vi "SPD.Get Meas pass and report.vi"(8 "error in (no error)":errorcluster, 11 "error or stoped":bool) -> (0 "error out":errorcluster, 2 "pass":bool, 3 "report":string)   [LabVIEW 2018]
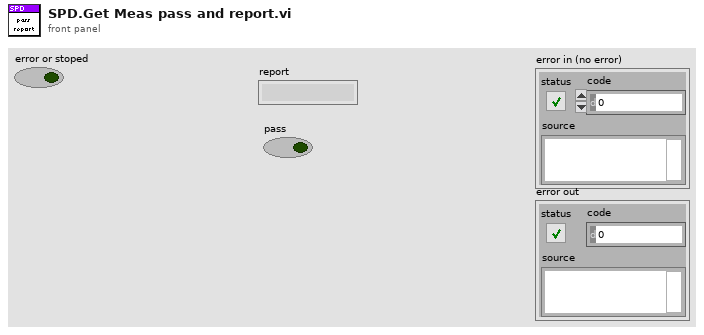
[diagram p1: front panel]
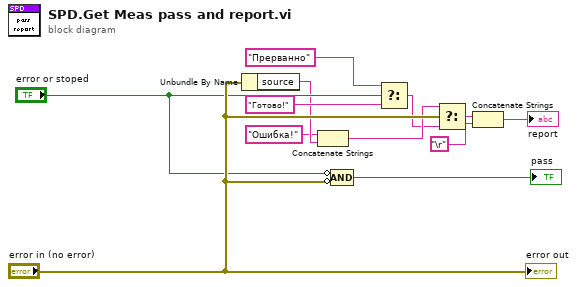
[diagram p0: block diagram]
diagram:
  n1 = Unbundle By Name("error in (no error)") -> ("source"=w5:string)
  n2 = Concatenate Strings("Ошибка!" ("t"), w5) -> (w4:string)
  n3 = Compound Arithmetic op=AND(invert "error or stoped", invert "error in (no error)") -> (→"pass":bool)
  n4 = Select(t="Прерванно" ("Report"), s="error or stoped", f="Готово!") -> (s? t:f=w2:string)
  n5 = Select(t=w4, s="error in (no error)", f=w2) -> (s? t:f=w7:string)
  n6 = Concatenate Strings(w7, "\r") -> (→"report":string)
  "error out" <- "error in (no error)"
